vi "SendPayLoad.vi"(8 "error in (no error)":errorcluster, 10 "PayLoad":T1[](array[typedef]) items=["Basic Control"=1, "Sound"=3, "Sound Sequence"=4, "Request Extra"=9, "General Purpose Output"=12, "Set Controller Gain"=13, "Get Controller Gain"=14], 11 "VISA Refnum in":refnum<visa-resource-name>) -> (0 "error out":errorcluster, 3 "VISA Refnum out":refnum<visa-resource-name>)   [LabVIEW 2018]
uses:
  Kobuki_cmdID.ctl
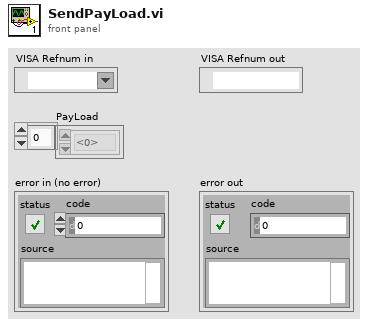
[diagram p1: front panel]
types:
  T1 = typedef "Kobuki_cmdID.ctl" = u8
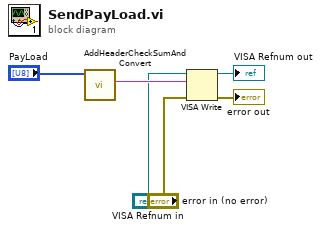
[diagram p0: block diagram]
diagram:
  n1 = call "AddHeaderCheckSumAndConvert.vi"("unsigned byte array"="PayLoad") -> ("string 2"=w4:string)  [unwired: 8 in, 2 out]
  n2 = VISA Write(VISA resource name="VISA Refnum in", write buffer=w4, error in (no error)="error in (no error)") -> (VISA resource name out=→"VISA Refnum out":refnum<visa-resource-name>, error out=→"error out":errorcluster)  [unwired: 1 out]
